vi "FUG-HCN.constructor.vi"(0 "name":string, 2 "data in":string, 5 "error in(no error)":errorcluster) -> (14 "i ref out":refnum<vi>, 16 "data out":string, 19 "error out":errorcluster)   [LabVIEW 2014, in "FUG-HCN.lvlib"]
doc: "High Voltage power supply FUG-HCN. This power supply can deliver upto 65KV. This class uses an instrument driver that is available via http://labview.gsi.de/driver.htm. The device is connected via GPIB. Finally, this device talks to a GPIB driver that must be installed on your system. Whenever a new frequency or amplitude value is set, that value is sent to the DSCInterface process for trending.\n\nauthors: Frank Herfurth (CERN) and Sumit Saxena\nadapted to CS v3 by: R.Savreux, CERN\n\nLicense Agreement for this software:\n\nCopyright (C)\nGesellschaft für Schwerionenforschung, GSI\nPlanckstr. 1\n64291 Darmstadt\nGermany\n\nContact: D.Beck@gsi.de \n\nThis program is free software; you can redistribute it and/or modify it under the terms of the \nGNU General Public License as published by the Free Software Foundation; either version 2 of \nthe license, or (at your option) any later version.\n\nThis program is distributed in the hope that it will be useful, but WITHOUT ANY WARRANTY; \nwithout even the implied warranty of MERCHANTABILITY or FITNESS FOR A PARTICULAR PURPOSE. See the GNU General License for more details (http://www.gnu.org).\n\nGesellschaft für Schwerionenforschung, GSI\nPlanckstr. 1, 64291 Darmstadt, Germany\nFor all questions and ideas contact: M.Richter@gsi.de, H.Brand@gsi.de or D.Beck@gsi.de.\nLast update: 16-JUN-2004"
uses:
  FUG-HCN.lvlib
  CSCore/BaseProcess/BaseProcess.lvlib
  CSCore/CSSystem/CSSystemLib/CSSystemLib.lvlib
  CSlibraries-extern/DimLVEvent/LVDimInterface/LVDimInterface.lvlib
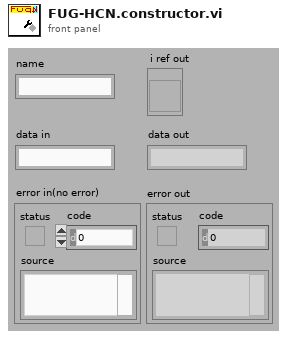
[diagram p1: front panel]
types:
  T1 = enum16{"SetAttribute", "GetAttribute", "CreateAttribute", "DestroyAttribute", "DestroyAllAtributes"}
  T2 = typedef "FUG-HCN.lvlib/FUG-HCN.i attribute.ctl" = cluster{"SetStatus":bool, "Set Voltage":dbl, "Nom Voltage":dbl, "VoltageID":i32, "CurrentID":i32}
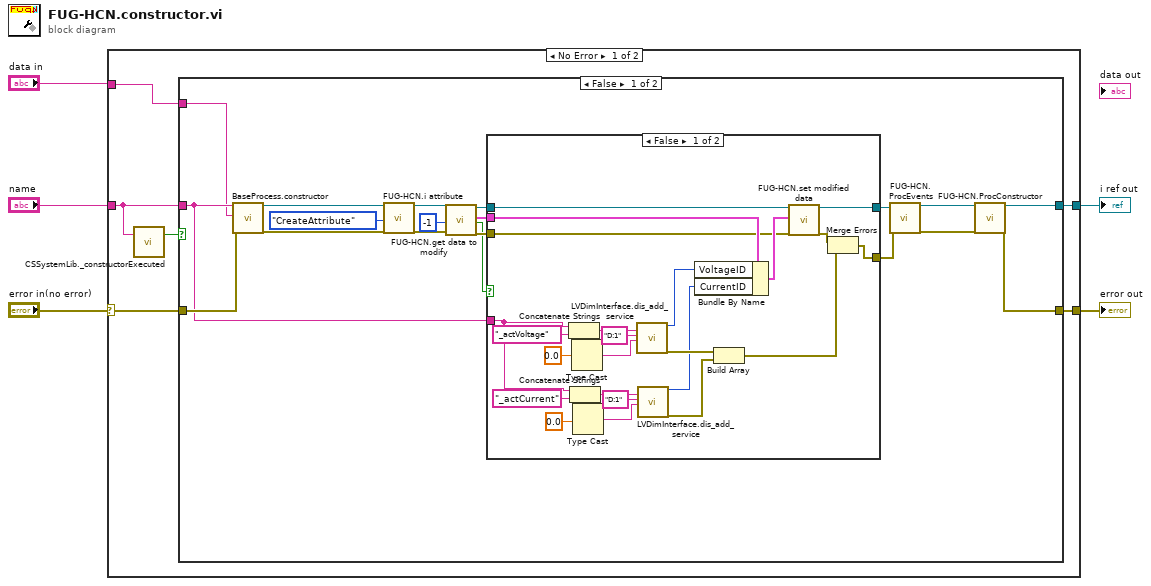
[diagram p0: block diagram]
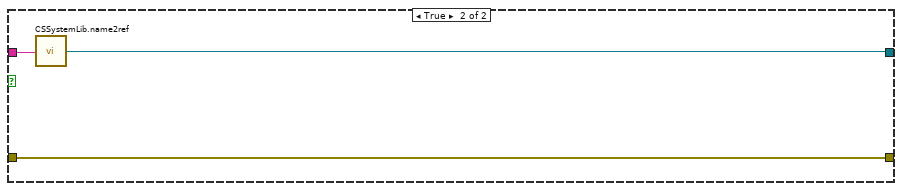
[diagram p3: hidden frame]
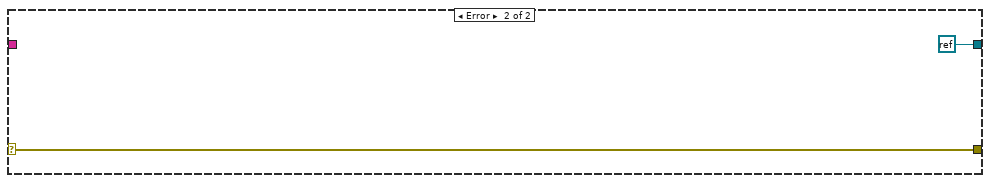
[diagram p4: hidden frame]
diagram:
  n1 = case shown="No Error" "error in(no error)" {
    selector: "error in(no error)" -> [w9 w60]
    tunnel: "name" -> [w8 _]
    tunnel: [w11 refnum<k0> refnum ("i ref out")] -> w4
    tunnel: [w10 w60] -> w3
    tunnel: "data in" -> [w6 _]
    frame No Error {
      n2 = call "CSSystemLib._constructorExecuted.vi"("name"=w8) -> ("constructor executed?"=w7:bool)  [unwired: 18 in]
      n3 = case shown="False" w7 {
        tunnel: [w25 w57] -> w11
        tunnel: [w24 w56] -> w10
        tunnel: w9 -> [w23 w56]
        tunnel: w8 -> [w13 w58]
        tunnel: w6 -> [w12 _]
        frame False {
          n4 = call "BaseProcess.constructor.vi"("name"=w13, "data in"=w12, "error in (no error)"=w23) -> ("i ref out"=w30:refnum<vi>, "error out"=w29:errorcluster)  [unwired: 14 in, 1 out]
          n5 = call "FUG-HCN.i attribute.vi"("VI Refnum"=w30, "Action"=T1."CreateAttribute", "error in (no error)"=w29) -> ("VI Refnum out"=w22:refnum<vi>, "error out"=w21:errorcluster)  [unwired: 14 in, 1 out]
          n6 = call "FUG-HCN.get data to modify.vi"("i ref in"=w22, "ms timeout (10000)"=-1, "error in (no error)"=w21) -> ("i ref out"=w18:refnum<vi>, "i attribute"=w19:T2, "timed out"=w14:bool, "error out"=w17:errorcluster)  [unwired: 13 in]
          n7 = case shown="False" w14 {
            tunnel: w19 -> [w51 _]
            tunnel: w18 -> [w50 w55]
            tunnel: w17 -> [w48 w54]
            tunnel: [w47 w55] -> w16
            tunnel: [w44 w54] -> w15
            tunnel: w13 -> [w31 _]
            frame False {
              n8 = Concatenate Strings(w31, "_actVoltage" ("string")) -> (w43:string)
              n9 = Concatenate Strings(w31, "_actCurrent" ("string")) -> (w41:string)
              n10 = Type Cast(x=0.0) -> (*(type *) &x=w42:string)  [unwired: 1 in]
              n11 = Type Cast(x=0.0) -> (*(type *) &x=w40:string)  [unwired: 1 in]
              n12 = call "LVDimInterface.dis_add_service.vi"("serviceName"=w43, "typeDescriptor"="D:1", "data"=w42) -> ("my_serviceID"=w33:i32, "error out"=w53:errorcluster)  [unwired: 15 in]
              n13 = call "LVDimInterface.dis_add_service.vi"("serviceName"=w41, "typeDescriptor"="D:1", "data"=w40) -> ("my_serviceID"=w32:i32, "error out"=w52:errorcluster)  [unwired: 15 in]
              n14 = Bundle By Name(cluster=w51, "VoltageID"=w33, "CurrentID"=w32) -> (w49:T2)
              n15 = Build Array(w53, w52) -> (w45:errorcluster[])
              n16 = call "FUG-HCN.set modified data.vi"("i ref in"=w50, "i attribute"=w49, "error in (no error)"=w48) -> ("i ref out"=w47:refnum<vi>, "error out"=w46:errorcluster)  [unwired: 15 in]
              n17 = Merge Errors(w46, w45) -> (w44:errorcluster)
            }
            frame True {
            }
          }
          n18 = call "FUG-HCN.ProcEvents.vi"("i ref in"=w16, "error in"=w15) -> ("i ref out"=w27:refnum<vi>, "error out"=w26:errorcluster)  [unwired: 16 in]
          n19 = call "FUG-HCN.ProcConstructor.vi"("i ref in"=w27, "error in (no error)"=w26) -> ("i ref out"=w25:refnum<vi>, "error out"=w24:errorcluster)  [unwired: 16 in]
        }
        frame True {
          n20 = call "CSSystemLib.name2ref.vi"("name"=w58) -> ("obj refnum"=w57:refnum<vi>)
        }
      }
    }
    frame Error {
    }
  }
  "i ref out" <- w4
  "error out" <- w3
